vi "Packed String to Variant.vi"(2 "Packed String":string, 4 "Type Descriptor":i16[](array[numeric]) format="%x") -> (5 "Variant":variant)   [LabVIEW 2018, in "Application.lvlib" / "Store.lvclass"]
uses:
  Store.lvclass
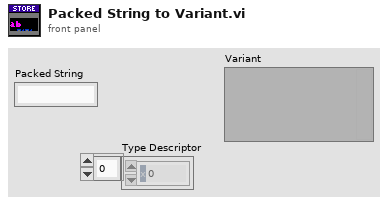
[diagram p1: front panel]
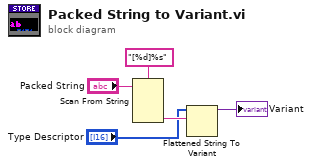
[diagram p0: block diagram]
diagram:
  n1 = Scan From String(format string="[%d]%s", input string="Packed String") -> (output 2=w3:string)  [unwired: 5 in, 3 out]
  n2 = Flattened String To Variant(6:w3, 7:"Type Descriptor") -> (3:→"Variant":variant)  [unwired: 1 in, 1 out]
